vi "Самолетт.vi"() -> ()   [LabVIEW 2021]
uses:
  Control 3.ctl
panel:
  in  "stop":bool
  in  "Plane":T1
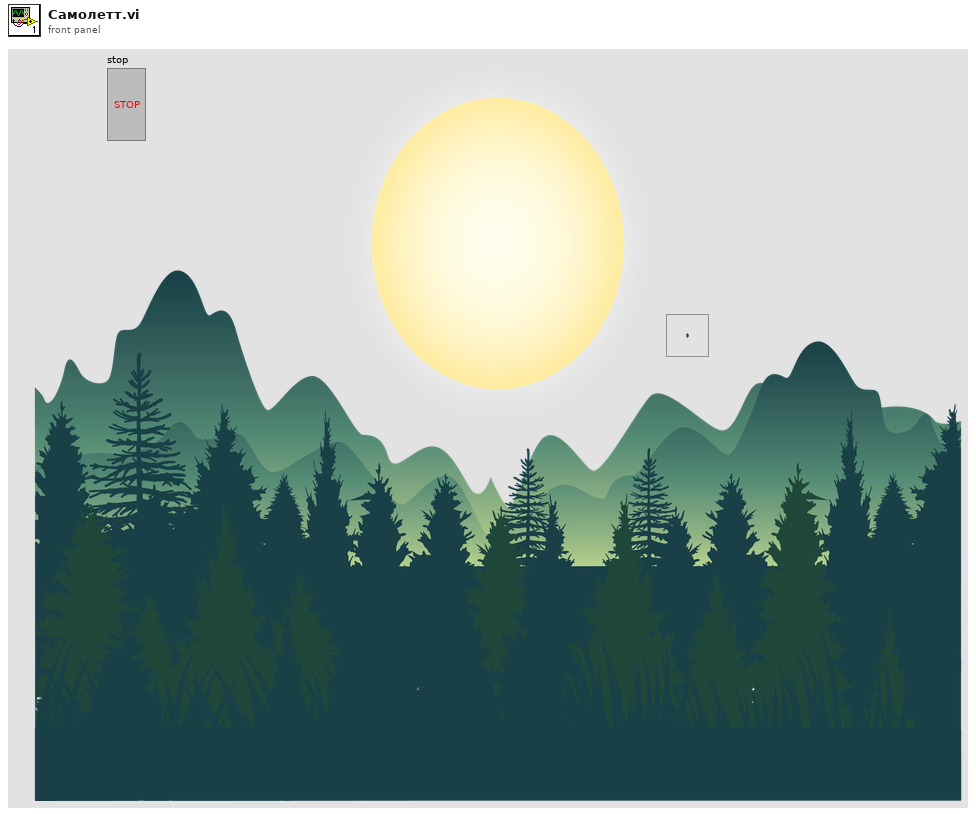
[diagram p1: front panel]
types:
  T1 = typedef "Control 3.ctl" = bool
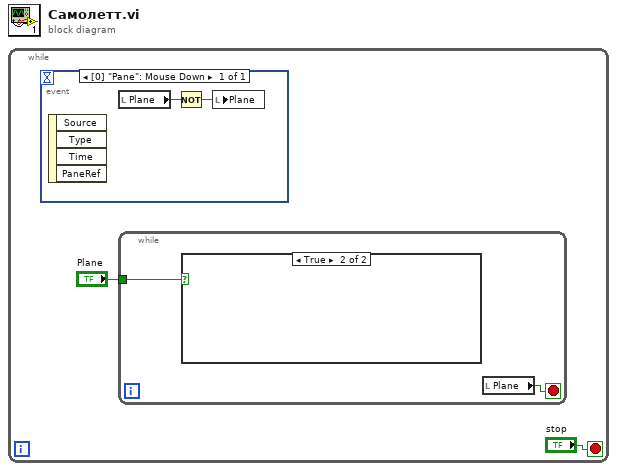
[diagram p0: block diagram]
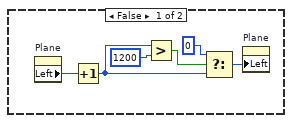
[diagram p2: hidden frame]
diagram:
  n1 = while {
    stop <- "stop" stop-if-true
    n2 = event shown="[0] \"Pane\": Mouse Down" {
      selector: _ -> [_]
      dyn-events: _ -> [_]
      timeout: _ -> [_]
      event Mouse Down {
        n3 = event-data() -> ()  [unwired: 1 in, 4 out]
        n4 = local read "Plane"() -> (w12:T1)
        n5 = Not(x=w12) -> (.not. x?=w11:T1)
        n6 = local write "Plane"(w11) -> ()
      }
    }
    n7 = while {
      tunnel: "Plane" -> [w4]
      stop <- w3 stop-if-true
      n8 = case shown="True" w4 {
        frame False {
          n9 = property on="Plane" class="Bool (strict)"() -> ("Left"=w10:i32)  [unwired: 2 in, 2 out]
          n10 = Increment(x=w10) -> (x+1=w8:i32)
          n11 = Greater?(x=w8, y=1200) -> (0:w9:bool)
          n12 = Select(t=0, s=w9, f=w8) -> (s? t:f=w7:i32)
          n13 = property on="Plane" class="Bool (strict)"("Left"=w7) -> ()  [unwired: 2 in, 2 out]
        }
        frame True {
        }
      }
      n14 = local read "Plane"() -> (w3:T1)
    }
  }
